vi "read_intercept_init.vi"(8 "error in (no error)":errorcluster, 11 "SGDRegressor in":refnum<class "SGDRegressor.lvclass">) -> (0 "error out":errorcluster, 2 "intercept_init":dbl[](array[numeric]), 3 "SGDRegressor out":refnum<class "SGDRegressor.lvclass">)   [LabVIEW 2020, in "SGDRegressor.lvclass"]
uses:
  SGDRegressor.lvclass
  SGDRegressor.lvclass/SGDRegressor.ctl
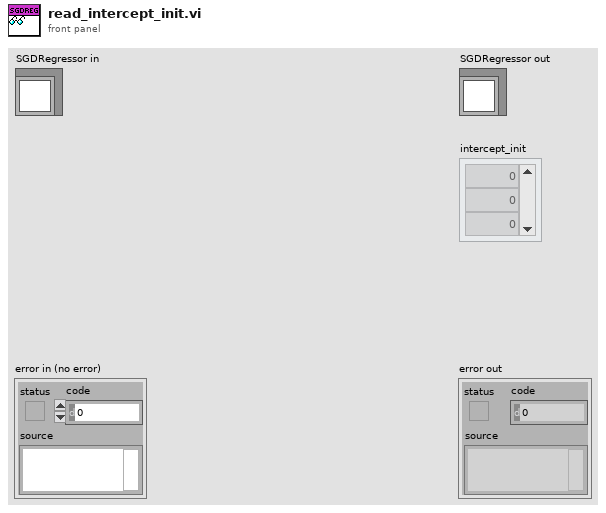
[diagram p1: front panel]
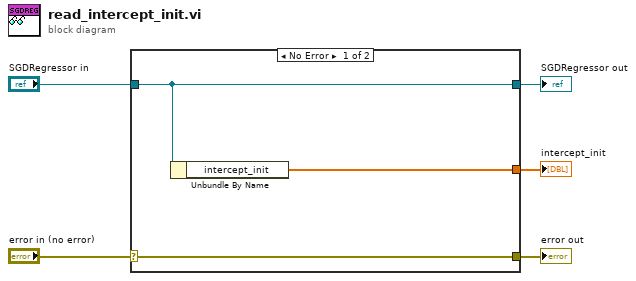
[diagram p0: block diagram]
diagram:
  n1 = case shown="No Error" "error in (no error)" {
    selector: "error in (no error)" -> [w8 w9]
    tunnel: [w8 w9] -> w4
    tunnel: [w7 w10] -> w2
    tunnel: "SGDRegressor in" -> [w7 w10]
    tunnel: [w6 _] -> w1
    frame No Error {
      n2 = Unbundle By Name(w7) -> ("intercept_init"=w6:dbl[])
    }
    frame Error {
    }
  }
  "error out" <- w4
  "SGDRegressor out" <- w2
  "intercept_init" <- w1
